vi "Set Weight Tool Vacuum.vi"(8 "error in":errorcluster, 9 "On/Off":bool, 11 "Gantry in":refnum<class "Gantry Class.lvclass">) -> (0 "error out":errorcluster, 3 "Gantry out":refnum<class "Gantry Class.lvclass">)   [LabVIEW 2011, in "Gantry Class.lvclass"]
uses:
  Gantry Class.lvclass
  WorkTable Class/WorkTable Class.lvclass
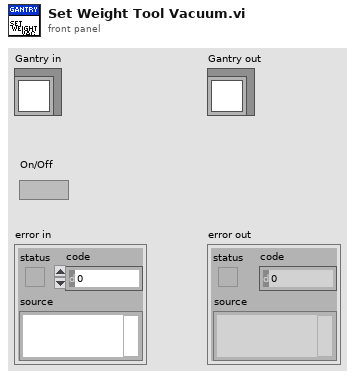
[diagram p1: front panel]
types:
  T1 = typedef "Worktable_Weights.ctl" = cluster{"Weight Slots":T2[], "Vacuum Channel":i32}
  T2 = typedef "Worktable_Weight.ctl" = cluster{"Weight State":enum16{"Empty", "Populated"}, "Weight Type":T3, "Location/Orientation":T4}
  T3 = typedef "Weight Type.ctl" = enum16{"Weight 1", "Weight 2", "Weight 3", "Weight 4", "Weight 5", "Weight 6", "Weight 7", "Weight 8"}
  T4 = typedef "Position_Orientation.ctl" = cluster{"Center":refnum<class "Vec3d Class.lvclass">, "Orientation":refnum<class "Orient3d Class.lvclass">}
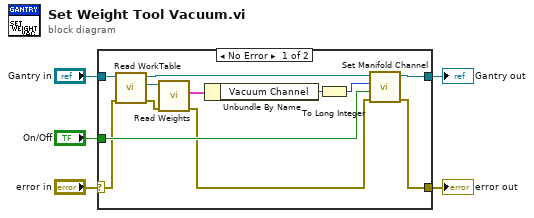
[diagram p0: block diagram]
diagram:
  n1 = case shown="No Error" "error in" {
    selector: "error in" -> [w9 w19]
    tunnel: [w13 w19] -> w2
    tunnel: [w14 w18] -> w3
    tunnel: "Gantry in" -> [w17 w18]
    tunnel: "On/Off" -> [w16 _]
    frame No Error {
      n2 = call-dynamic "Read WorkTable.vi"("error in"=w9, "Gantry Class in"=w17) -> ("error out"=w10:errorcluster, "WorkTable Class.lvclass"=w12:refnum<class "WorkTable Class.lvclass">, "Gantry Class out"=w15:refnum<class "Gantry Class.lvclass">)  [unwired: 7 in]
      n3 = call-dynamic "Read Weights.vi"("error in (no error)"=w10, "WorkTable Class in"=w12) -> ("error out"=w8:errorcluster, "Weights"=w11:T1)  [unwired: 7 in, 1 out]
      n4 = Unbundle By Name(w11) -> ("Vacuum Channel"=w7:i32)
      n5 = To Long Integer(number=w7) -> (32bit integer=w6:i32)
      n6 = call-dynamic "Set Manifold Channel.vi"("error in"=w8, "On/Off"=w16, "Manifold Channel"=w6, "Gantry in"=w15) -> ("error out"=w13:errorcluster, "Gantry out"=w14:refnum<class "Gantry Class.lvclass">)  [unwired: 6 in]
    }
    frame Error {
    }
  }
  "error out" <- w2
  "Gantry out" <- w3
